vi "Rename State Calls.vi"(8 "error in (no error)":errorcluster, 9 "New State Name":string, 10 "Old State Name":string, 11 "JKI SM in":refnum<class "JKI SM.lvclass">) -> (0 "error out":errorcluster, 3 "JKI SM out":refnum<class "JKI SM.lvclass">)   [LabVIEW 2020, in "JKI State Machine API.lvlib" / "JKI SM.lvclass"]
uses:
  JKI SM.lvclass
  <vilib>/Utility/traverseref.llb/TRef TravTarget.ctl
  JKI SM.lvclass/JKI SM.ctl
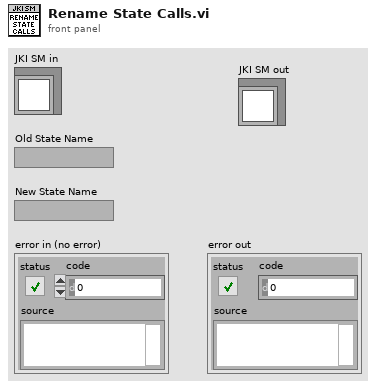
[diagram p1: front panel]
types:
  T1 = typedef "TRef TravTarget.ctl" = enum16{"FP", "BD", "Other"}
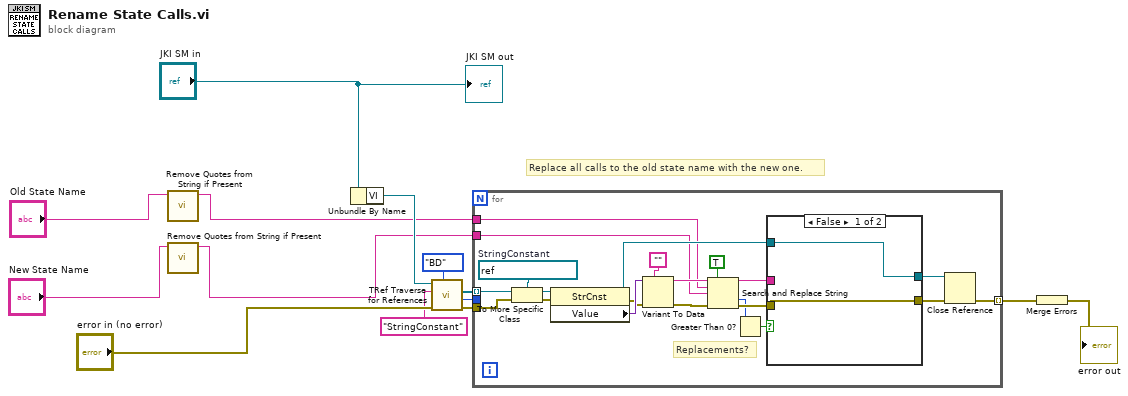
[diagram p0: block diagram]
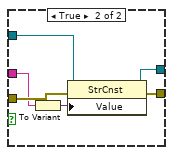
[diagram p2: hidden frame]
diagram:
  # "Replace all calls to the old state name with the new one."
  n1 = call "Remove Quotes from String if Present.vi"("String"="Old State Name") -> ("String with Quotes Removed"=w3:string)  [unwired: 10 in]
  n2 = call "Remove Quotes from String if Present.vi"("String"="New State Name") -> ("String with Quotes Removed"=w1:string)  [unwired: 10 in]
  n3 = Unbundle By Name("JKI SM in") -> ("VI"=w6:refnum<vi>)
  n4 = call <vilib>:"TRef Traverse for References.vi"("Traverse Target"=TRef_TravTarget."BD", "error in (no error)"="error in (no error)", "Class Name"="StringConstant", "VI Refnum"=w6) -> ("error out"=w7:errorcluster, "# of Refs"=w14:i32, "References"=w8:refnum<vi>[])  [unwired: 1 in, 4 out]
  n5 = for {
    tunnel: w8 -> [w35] mode=indexing
    tunnel: w7 -> [w32]
    tunnel: w3 -> [w19]
    tunnel: w1 -> [w18]
    tunnel: [w21] -> w11 mode=indexing
    tunnel: w14 -> [_]
    w33 = refnum<vi> refnum  # StringConstant
    # "Replacements?"
    n6 = To More Specific Class(target class=w33, reference=w35, error in=w32) -> (specific class reference=w34:refnum<vi>, error out=w31:errorcluster)
    n7 = property class="StrCnst"(reference=w34, error in=w31) -> (reference out=w24:refnum<vi>, error out=w27:errorcluster, "Value"=w30:variant)
    n8 = Variant To Data(error in=w27, type="", Variant=w30) -> (data=w20:string, error out=w28:errorcluster)
    n9 = Search and Replace String(replace all?=TRUE ("replace all? (F)"), input string=w20, search string=w19, replace string=w18, error in=w28) -> (result string=w17:string, offset past replacement=w16:i32, error out=w25:errorcluster)  [unwired: 3 in, 1 out]
    n10 = Greater Than 0?(x=w16) -> (x > 0?=w15:bool)
    n11 = case shown="False" w15 {
      tunnel: w25 -> [w36 w43]
      tunnel: w24 -> [w37 w42]
      tunnel: [w36 w40] -> w23
      tunnel: [w37 w39] -> w22
      tunnel: w17 -> [_ w38]
      frame False {
      }
      frame True {
        n12 = To Variant(anything=w38) -> (Variant=w41:variant)
        n13 = property class="StrCnst"(reference=w42, error in=w43, "Value"=w41) -> (reference out=w39:refnum<vi>, error out=w40:errorcluster)
      }
    }
    n14 = Close Reference(reference=w22, error in (no error)=w23) -> (error out=w21:errorcluster)
  }
  n15 = Merge Errors(w11) -> (→"error out":errorcluster)
  "JKI SM out" <- "JKI SM in"
